vi "Arrange VIWin - Get Window Gaps.vi"(0 "window type":T1, 11 "error in":errorcluster) -> (4 "window gaps":T2, 15 "error out":errorcluster)   [LabVIEW 2014, in "Arrange VI Window.lvlib"]
uses:
  Arrange VI Window.lvlib
  Arrange VIWin - Window Gaps.ctl
  Arrange VIWin - Window Type.ctl
  <resource>/dialog/lvconfig.llb/LV Config Read Numeric (I32).vi
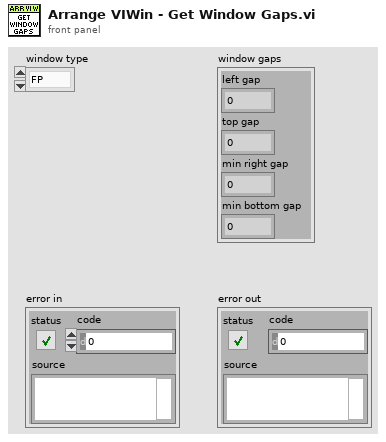
[diagram p1: front panel]
types:
  T1 = typedef "Arrange VI Window.lvlib/Arrange VIWin - Window Type.ctl" = enum16{"FP", "BD"}
  T2 = typedef "Arrange VI Window.lvlib/Arrange VIWin - Window Gaps.ctl" = cluster{"left gap":i16, "top gap":i16, "min right gap":i16, "min bottom gap":i16}
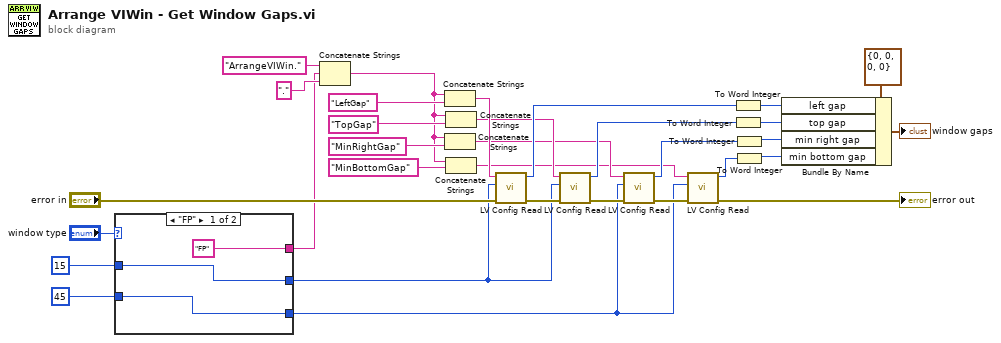
[diagram p0: block diagram]
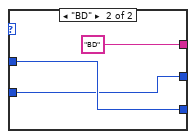
[diagram p2: hidden frame]
diagram:
  n1 = case shown="\"FP\"" "window type" {
    tunnel: ["FP" "BD"] -> w13
    tunnel: [w33 w37] -> w3
    tunnel: 15 -> [w34 w37]
    tunnel: [w34 w36] -> w1
    tunnel: 45 -> [w33 w36]
    frame "FP" {
    }
    frame "BD" {
    }
  }
  n2 = Concatenate Strings("ArrangeVIWin." ("string"), w13, "." ("string")) -> (w8:string)
  n3 = Concatenate Strings(w8, "LeftGap" ("key")) -> (w12:string)
  n4 = Concatenate Strings(w8, "MinRightGap" ("key")) -> (w6:string)
  n5 = Concatenate Strings(w8, "TopGap" ("key")) -> (w7:string)
  n6 = Concatenate Strings(w8, "MinBottomGap" ("key")) -> (w5:string)
  n7 = call-poly <resource>:"LV Config Read.vi"("error in"="error in", "default value"=w1, "key"=w12) -> ("error out"=w31:errorcluster, "value"=w30:i32)  [unwired: 2 in, 1 out]
  n8 = call-poly <resource>:"LV Config Read.vi"("error in"=w31, "default value"=w1, "key"=w7) -> ("error out"=w24:errorcluster, "value"=w23:i32)  [unwired: 2 in, 1 out]
  n9 = call-poly <resource>:"LV Config Read.vi"("error in"=w24, "default value"=w3, "key"=w6) -> ("error out"=w22:errorcluster, "value"=w18:i32)  [unwired: 2 in, 1 out]
  n10 = call-poly <resource>:"LV Config Read.vi"("error in"=w22, "default value"=w3, "key"=w5) -> ("error out"=→"error out":errorcluster, "value"=w21:i32)  [unwired: 2 in, 1 out]
  n11 = To Word Integer(number=w30) -> (16bit integer=w28:i16)
  n12 = To Word Integer(number=w23) -> (16bit integer=w27:i16)
  n13 = To Word Integer(number=w18) -> (16bit integer=w19:i16)
  n14 = To Word Integer(number=w21) -> (16bit integer=w20:i16)
  n15 = Bundle By Name(cluster=T2 {"left gap"=0, "top gap"=0, "min right gap"=0, "min bottom gap"=0} ("Display:Primary Workspace"), "left gap"=w28, "top gap"=w27, "min right gap"=w19, "min bottom gap"=w20) -> (→"window gaps":T2)
